vi "flat_secuence_bloqueante}.vi"() -> ()   [LabVIEW 2020]
panel:
  out "Boolean":bool
  in  "Button":bool
  out "Tank 4":u8(slide) scale=0.0..100.0
  in  "stop":bool
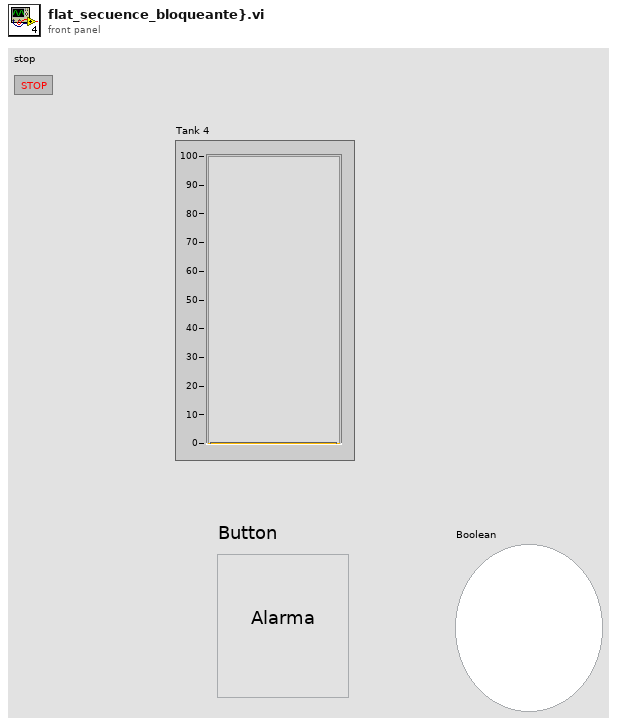
[diagram p1: front panel]
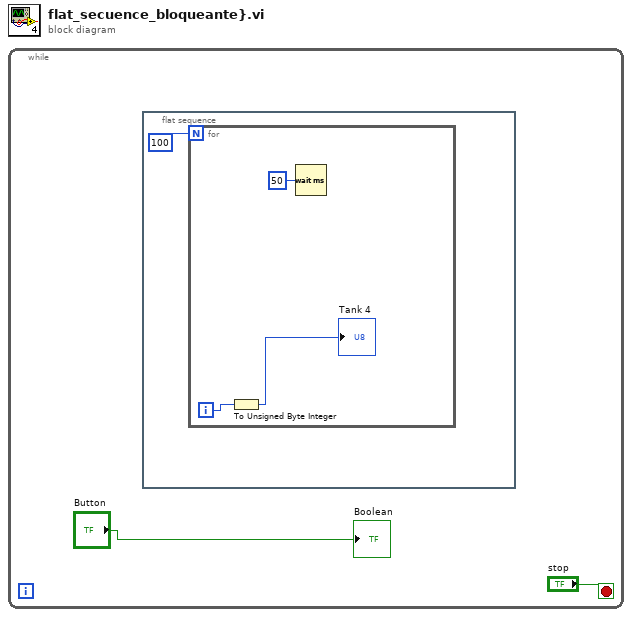
[diagram p0: block diagram]
diagram:
  n1 = while {
    stop <- "stop" stop-if-true
    n2 = flat-sequence {
      frame #0 {
        n3 = for {
          N: 100 -> [_]
          i -> [w6]
          n4 = To Unsigned Byte Integer(number=w6) -> (unsigned 8bit integer=→"Tank 4":u8)
          n5 = Wait (ms)(milliseconds to wait=u32 50) -> ()  [unwired: 1 out]
        }
      }
    }
    "Boolean" <- "Button"
  }
